vi "市电监测-自动重合闸.vi"() -> ()   [LabVIEW 2016, in "环境动力监测库.lvlib" / "自动重合闸库.lvlib"]
uses:
  <vilib>/Utility/miscctls.llb/LVPointTypeDef.ctl
  <vilib>/ptbypt/NI_PtbyPt.lvlib
  <vilib>/Utility/config.llb/NI_LVConfig.lvlib
panel:
  in  "解除告警":bool
  out "日用电量":dbl caption="日用电量：" format="%#.1f"
  out "小时用电量":dbl caption="小时用电量：" format="%#.1f"
  in  "清零":bool
  out "累计用电量":dbl caption="累计用电量：" format="%#.1f"
  out "漏电报警累加值":u16 caption="漏电报警次数："
  out "当前报警状态":u16(ring) caption="当前报警状态：" items=["无报警"=0, "过压报警"=1, "欠压报警"=2, "过流报警"=4, "漏电报警"=8]
  out "通讯状态":u16(ring) caption="通讯状态：" items=["正常", "异常"]
  out "过流报警累加值":u16 caption="过流报警次数："
  out "欠压报警累加值":u16 caption="欠压报警次数："
  out "过压报警累加值":u16 caption="过压报警次数："
  out "当前漏电电流":dbl caption="当前漏电电流："
  out "当前电流":dbl caption="当前电流："
  out "当前电压":u16 caption="当前电压："
  # "市电监测/自动重合闸"
  # "KW·h"
  # "KW·h"
  # "KW·h"
  # "mA"
  # "A"
  # "V"
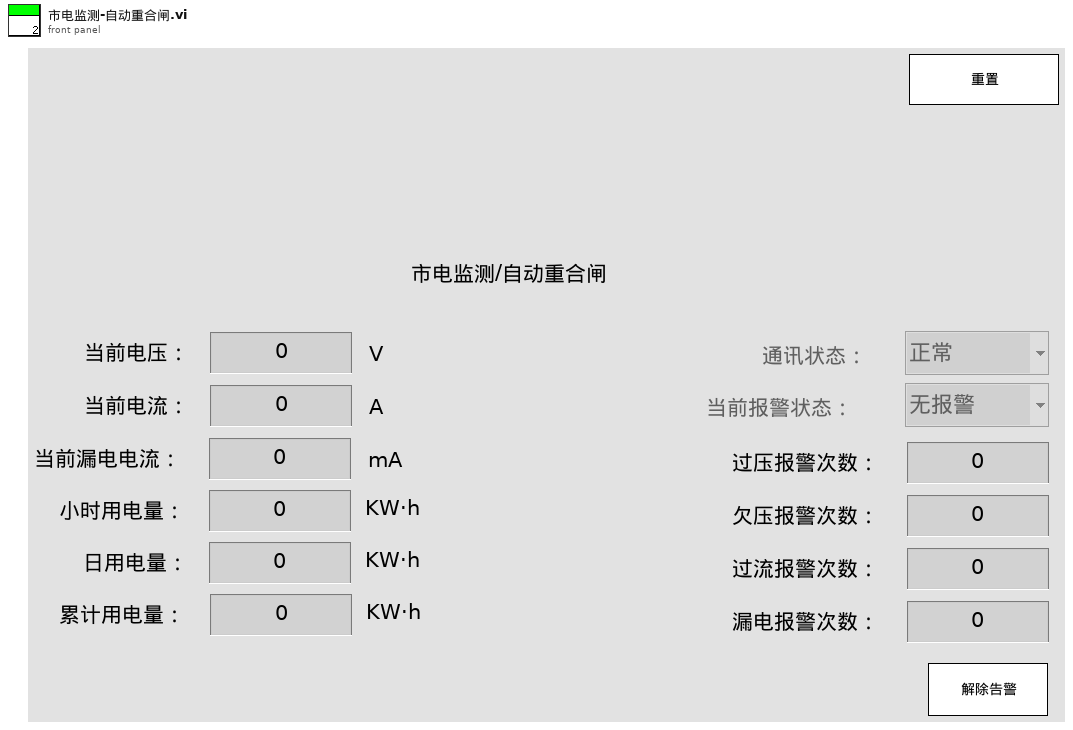
[diagram p1: front panel]
types:
  T1 = typedef "LVPointTypeDef.ctl" = cluster{"Horizontal":i16, "Vertical":i16}
  T2 = typedef "NI_LVConfig.lvlib/Config Data RefNum.ctl" = refnum<k1>
  T3 = cluster{"时间标识":timestamp, "设备":string, "日志信息":string}
  T4 = cluster{"状态":cluster{"R0":i16, "R1":i16, "R2":i16, "R3":i16, "R4":i16, "R5":i16, "R6":i16, "R7":i16, "R8":i16, "R9":i16, "R10":i16, "R11":i16, "R12":i16, "R13":i16, "R14":i16, "R15":i16, "R16":i16, "R17":i16, "R18":i16, "R19":i16, "R20":i16, "R21":i16, "R22":i16, "R23":i16, "R24":i16, "R25":i16, "R26":i16, "R27":i16, "R28":i16, "R29":i16, "R30":i16, "R31":i16, "R32":i16, "R33":i16, "R34":i16, "R35":i16, "R36":i16, "R37":i16, "R38":i16, "R39":i16}, "输入状态":bool[], "输出状态":bool[], "参数设置":cluster{"R100":i16, "R101":i16, "R102":i16, "R103":i16, "R104":i16, "R105":i16, "R106":i16, "R107":i16, "R108":i16, "R109":i16, "R110":i16, "R111":i16, "R112":i16, "R113":i16, "R114":i16, "R115":i16, "R116":i16, "R117":i16, "R118":i16, "R119":i16, "R120":i16, "R121":i16, "R122":i16, "R123":i16}, "转换值":cluster{"AD0":sgl, "AD1":sgl, "AD2":sgl, "AD3":sgl, "AD4":sgl, "AD5":sgl}}
  T5 = cluster{"R0":i16, "R1":i16, "R2":i16, "R3":i16, "R4":i16, "R5":i16, "R6":i16, "R7":i16, "R8":i16, "R9":i16, "R10":i16, "R11":i16, "R12":i16, "R13":i16, "R14":i16, "R15":i16, "R16":i16, "R17":i16, "R18":i16, "R19":i16, "R20":i16, "R21":i16, "R22":i16, "R23":i16, "R24":i16, "R25":i16, "R26":i16, "R27":i16, "R28":i16, "R29":i16, "R30":i16, "R31":i16, "R32":i16, "R33":i16, "R34":i16, "R35":i16, "R36":i16, "R37":i16, "R38":i16, "R39":i16}
  T6 = cluster{"状态":cluster{"R0":i16, "R1":i16, "R2":i16, "R3":i16, "R4":i16, "R5":i16, "R6":i16, "R7":i16, "R8":i16, "R9":i16, "R10":i16, "R11":i16, "R12":i16, "R13":i16, "R14":i16, "R15":i16, "R16":i16, "R17":i16, "R18":i16, "R19":i16, "R20":i16, "R21":i16, "R22":i16, "R23":i16, "R24":i16, "R25":i16, "R26":i16, "R27":i16, "R28":i16, "R29":i16, "R30":i16, "R31":i16, "R32":i16, "R33":i16, "R34":i16, "R35":i16, "R36":i16, "R37":i16, "R38":i16, "R39":i16, "R40":i16, "R41":i16, "R42":i16, "R43":i16, "R44":i16, "R45":i16, "R46":i16, "R47":i16, "R48":i16, "R49":i16, "R50":i16, "R51":i16, "R52":i16, "R53":i16, "R54":i16, "R55":i16, "R56":i16, "R57":i16, "R58":i16, "R59":i16, "R60":i16, "R61":i16, "R62":i16, "R63":i16, "R64":i16, "R65":i16, "R66":i16, "R67":i16, "R68":i16, "R69":i16}, "输入状态":bool[], "输出状态":bool[], "报警簇":bool[], "参数设置":cluster{"R100":i16, "R101":i16, "R102":i16, "R103":i16, "R104":i16, "R105":i16, "R106":i16, "R107":i16, "R108":i16, "R109":i16, "R110":i16, "R111":i16, "R112":i16, "R113":i16, "R114":i16, "R115":i16, "R116":i16, "R117":i16, "R118":i16, "R119":i16, "R120":i16, "R121":i16, "R122":i16, "R123":i16, "R124":i16}, "转换值":cluster{"AD0":sgl, "AD1":sgl, "AD2":sgl, "AD3":sgl, "AD4":sgl, "AD5":sgl}, "看门狗启用":bool, "氨氮模块名称":string, "总磷模块名称":string}
  T7 = cluster{"R0":i16, "R1":i16, "R2":i16, "R3":i16, "R4":i16, "R5":i16, "R6":i16, "R7":i16, "R8":i16, "R9":i16, "R10":i16, "R11":i16, "R12":i16, "R13":i16, "R14":i16, "R15":i16, "R16":i16, "R17":i16, "R18":i16, "R19":i16, "R20":i16, "R21":i16, "R22":i16, "R23":i16, "R24":i16, "R25":i16, "R26":i16, "R27":i16, "R28":i16, "R29":i16, "R30":i16, "R31":i16, "R32":i16, "R33":i16, "R34":i16, "R35":i16, "R36":i16, "R37":i16, "R38":i16, "R39":i16, "R40":i16, "R41":i16, "R42":i16, "R43":i16, "R44":i16, "R45":i16, "R46":i16, "R47":i16, "R48":i16, "R49":i16, "R50":i16, "R51":i16, "R52":i16, "R53":i16, "R54":i16, "R55":i16, "R56":i16, "R57":i16, "R58":i16, "R59":i16, "R60":i16, "R61":i16, "R62":i16, "R63":i16, "R64":i16, "R65":i16, "R66":i16, "R67":i16, "R68":i16, "R69":i16}
  T8 = cluster{"漏水监测输出":cluster{"漏水监测告警":bool, "告警内容":string}, "门禁监测输出":cluster{"门禁监测告警":bool, "告警内容":string}, "门禁监测输出2":cluster{"门禁监测告警":bool, "告警内容":string}, "温湿度监测输出":cluster{"温湿度监测告警":bool, "告警内容":string}, "烟雾监测输出":cluster{"烟雾监测告警":bool, "告警内容":string}, "空调监测输出":cluster{"空调监测告警":bool, "告警内容":string}, "自动重合闸输出":cluster{"自动重合闸告警":bool, "告警内容":string}, "红外入侵输出":cluster{"红外入侵告警":bool, "告警内容":string}, "振动输出":cluster{"振动告警":bool, "告警内容":string}, "UPS输出":cluster{"UPS告警":bool, "告警内容":string}, "蓄电池输出":cluster{"蓄电池告警":bool, "告警内容":string}, "蓄电池输出2":cluster{"蓄电池告警":bool, "告警内容":string}, "GPS输出":cluster{"定位告警":bool, "告警内容":string}, "北斗输出":cluster{"定位告警":bool, "告警内容":string}, "气象输出":cluster{"气象告警":bool, "告警内容":string}}
  T9 = cluster{"市电":cluster{"状态":bool, "电压:":u16, "电流：":dbl, "详情  ":bool}, "UPS":cluster{"状态":bool, "输入电压:":sgl, "输出电压:":sgl, "电池电量:":u8, "电量":u16, "详情  ":bool}, "蓄电池12V":cluster{"状态":bool, "电压:":sgl, "电流:":sgl, "电池电量:":u8, "电量":u16, "详情  ":bool}, "蓄电池24V":cluster{"状态":bool, "电压:":sgl, "电流:":sgl, "电池电量:":u8, "电量":u16, "详情  ":bool}}
  T10 = cluster{"时间标识":timestamp, "测量模式":string, "数据类型":string, "监测值":sgl, "单位":string, "数据标识":string, "因子编码":string}
  T11 = typedef "LVDateTimeRec.ctl" = cluster{"秒数的小数部分":dbl, "秒":i32, "分":i32, "时":i32, "日":i32, "月":i32, "年":i32, "天数（周）":i32, "天数（年）":i32, "DST":i32}
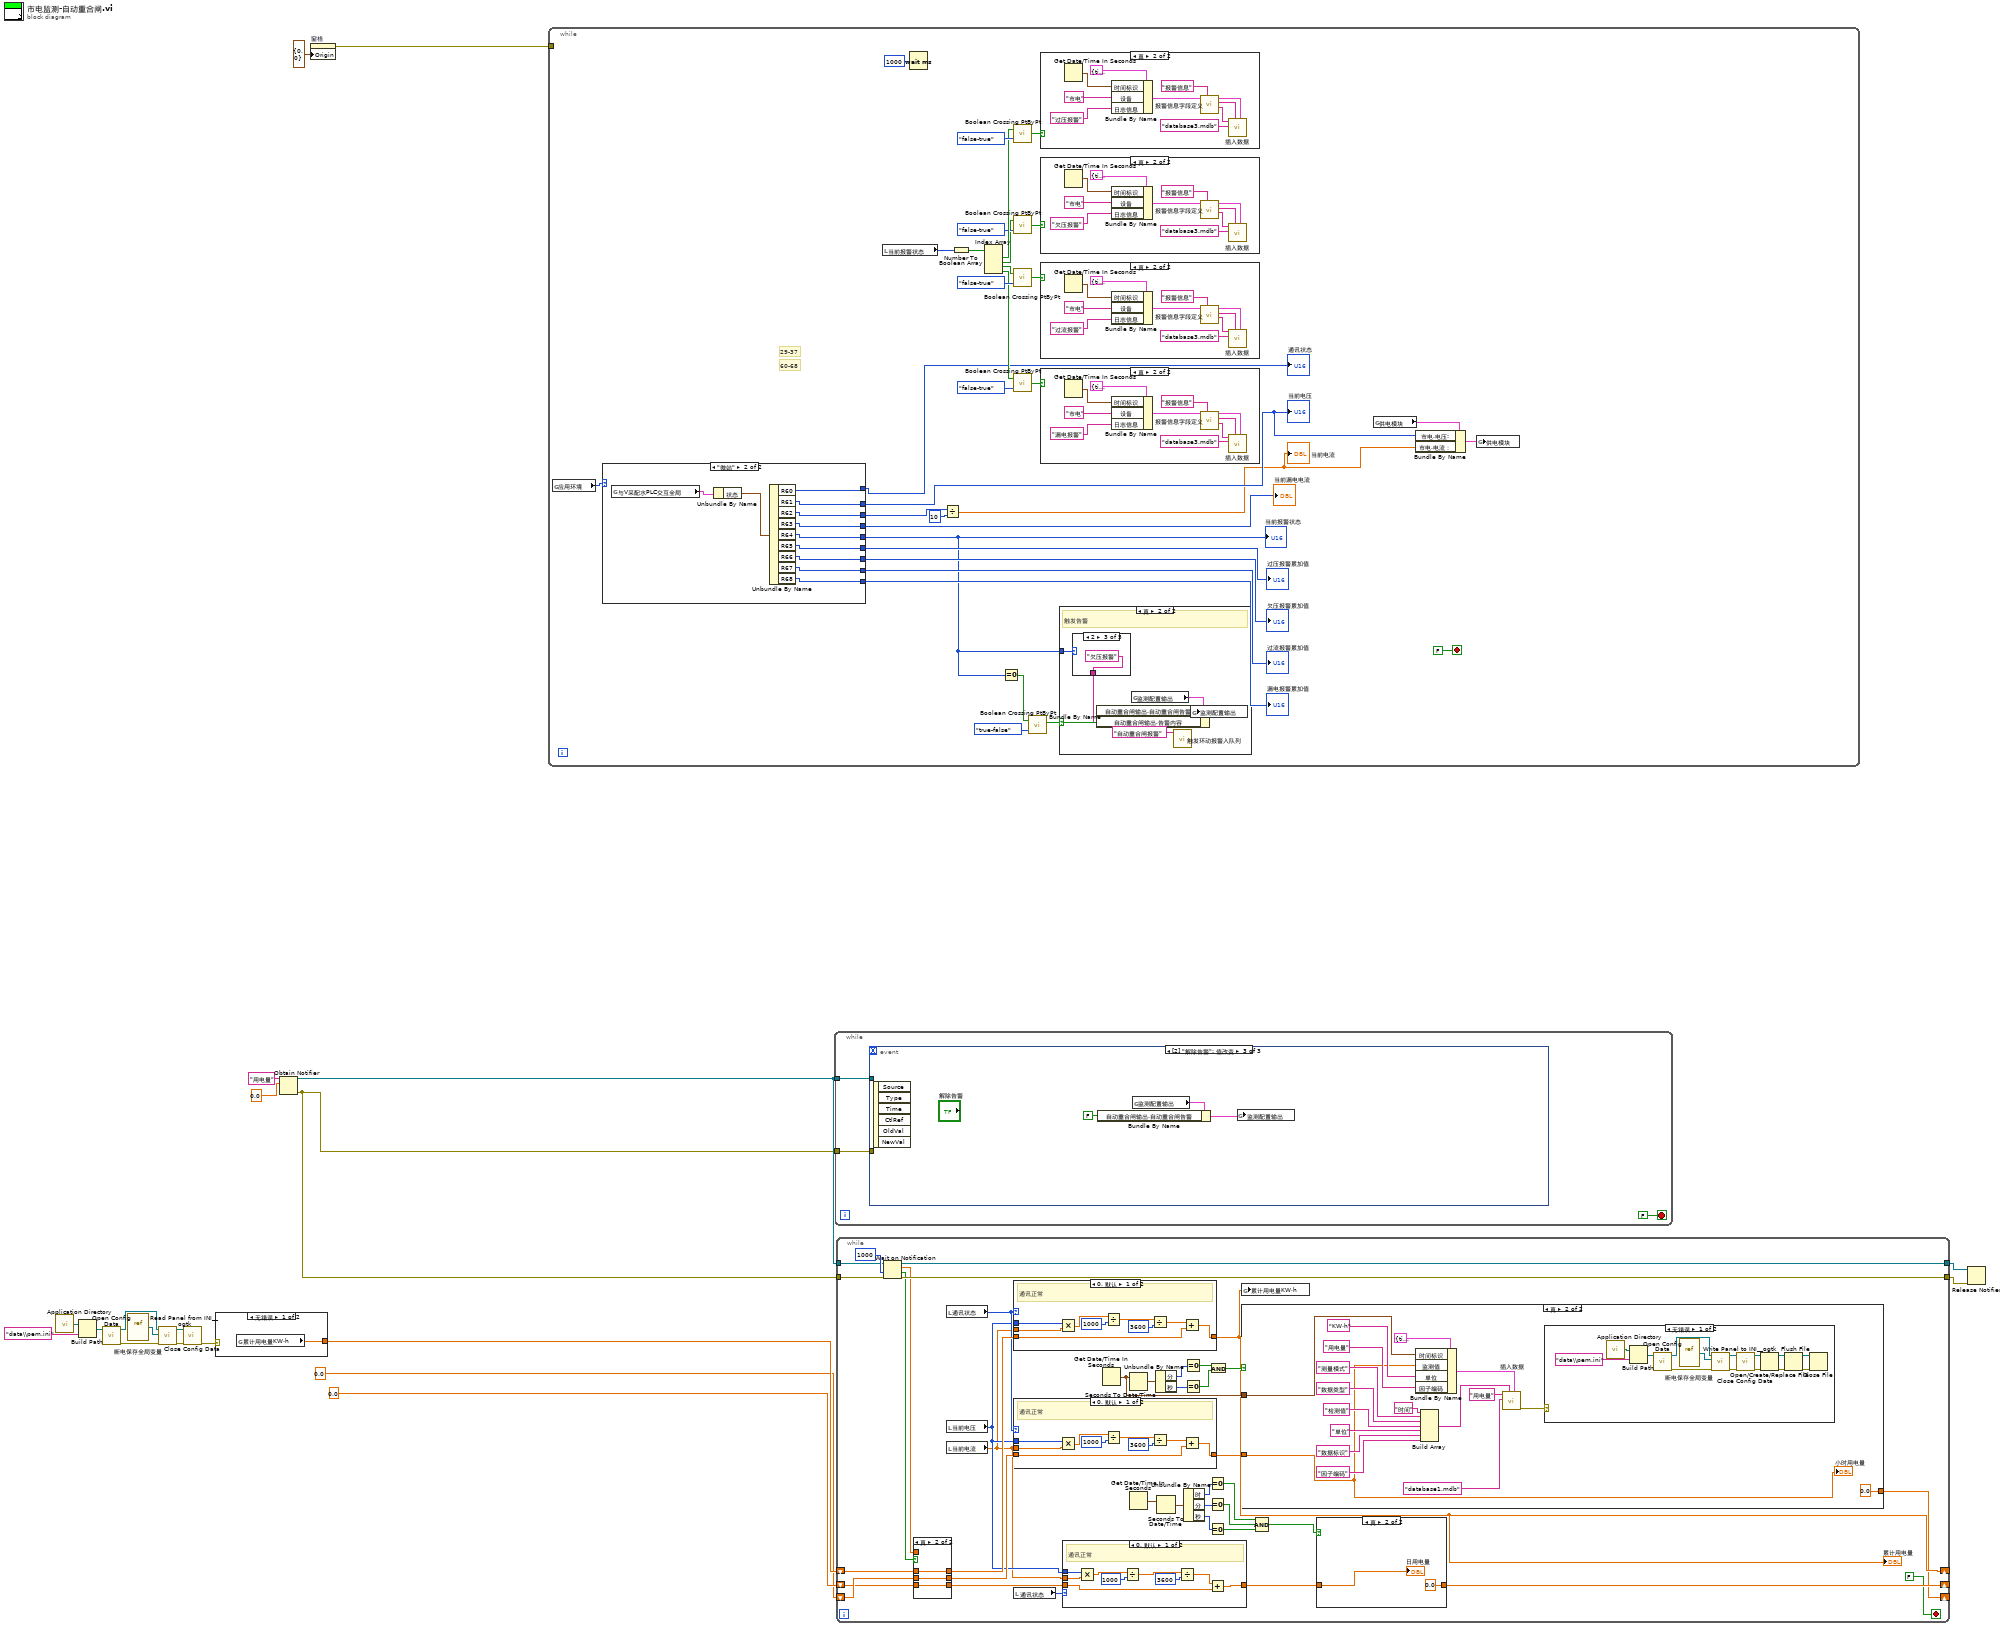
[diagram p0: block diagram]
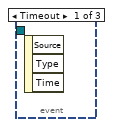
[diagram p9: hidden frame]
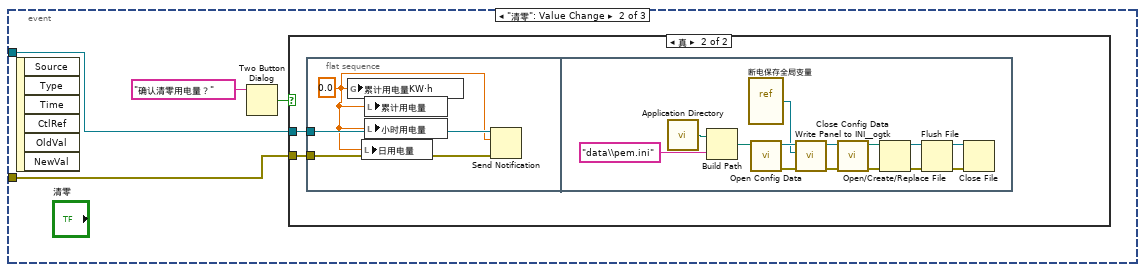
[diagram p10: hidden frame]
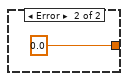
[diagram p12: hidden frame]
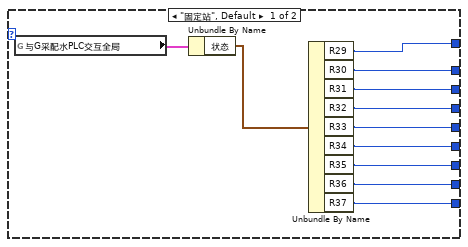
[diagram p13: hidden frame]
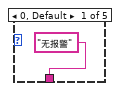
[diagram p15: hidden frame]
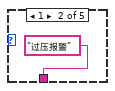
[diagram p16: hidden frame]
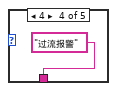
[diagram p17: hidden frame]
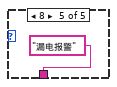
[diagram p18: hidden frame]
diagram:
  n1 = call <vilib>:"Application Directory.vi"() -> ("Application Directory"=w18:path)
  n2 = Build Path(base path=w18, name or relative path="data\\pem.ini" ("名称或相对路径")) -> (appended path=w16:path)
  n3 = call <vilib>:"Open Config Data.vi"("configuration file path"=w16) -> ("error out"=w12:errorcluster, "refnum"=w15:T2)  [unwired: 8 in, 1 out]
  n4 = vi-ref "断电保存全局变量.vi"() -> (w14:refnum<vi>)
  n5 = call <userlib>:"Read Panel from INI__ogtk.vi"("error in (no error)"=w12, "VI ref"=w14, "refnum"=w15) -> ("error out"=w11:errorcluster, "refnum out"=w13:T2)  [unwired: 7 in]
  n6 = call <vilib>:"Close Config Data.vi"("error in (no error)"=w11, "refnum"=w13) -> ("error out"=w10:errorcluster)  [unwired: 8 in, 1 out]
  n7 = case shown="无错误" w10 {
    tunnel: [w21 0.0 ("累计用电量KW/h")] -> w3
    frame No Error {
      n8 = global read "断电保存全局变量.vi" "累计用电量KW·h"() -> (w21:dbl)
    }
    frame Error {
    }
  }
  n9 = Obtain Notifier(name (unnamed)="用电量" ("名称（未命名）"), notification data type=0.0 ("y")) -> (notifier out=w7:refnum<notifier>, error out=w6:errorcluster)  [unwired: 2 in, 1 out]
  n10 = property on="窗格" class="Pane"("Origin"=T1 {"Horizontal"=0, "Vertical"=0} ("原点")) -> (error out=w19:errorcluster)  [unwired: 2 in, 1 out]
  n11 = while {
    tunnel: w19 -> [_]
    stop <- FALSE stop-if-true
    # "60-68"
    # "29-37"
    n12 = global read "外部交互全局变量.vi" "应用环境"() -> (w36:enum16{"固定站", "微站", "浮标", "浮船"})
    n13 = case shown="\"微站\"" w36 {
      tunnel: [w64 w75] -> w35
      tunnel: [w63 w74] -> w25
      tunnel: [w62 w73] -> w34
      tunnel: [w61 w72] -> w33
      tunnel: [w60 w71] -> w23
      tunnel: [w59 w70] -> w32
      tunnel: [w58 w69] -> w31
      tunnel: [w57 w68] -> w30
      tunnel: [w56 w67] -> w29
      frame "固定站", Default {
        n14 = global read "外部交互全局变量.vi" "与G采配水PLC交互全局"() -> (w66:T4)
        n15 = Unbundle By Name(w66) -> ("状态"=w65:T5)
        n16 = Unbundle By Name(w65) -> ("R29"=w64:i16, "R30"=w63:i16, "R31"=w62:i16, "R32"=w61:i16, "R33"=w60:i16, "R34"=w59:i16, "R35"=w58:i16, "R36"=w57:i16, "R37"=w56:i16)
      }
      frame "微站" {
        n17 = global read "外部交互全局变量.vi" "与V采配水PLC交互全局"() -> (w77:T6)
        n18 = Unbundle By Name(w77) -> ("状态"=w76:T7)
        n19 = Unbundle By Name(w76) -> ("R60"=w75:i16, "R61"=w74:i16, "R62"=w73:i16, "R63"=w72:i16, "R64"=w71:i16, "R65"=w70:i16, "R66"=w69:i16, "R67"=w68:i16, "R68"=w67:i16)
      }
    }
    "通讯状态" <- w35
    "当前电压" <- w25
    "当前漏电电流" <- w33
    "当前报警状态" <- w23
    "过压报警累加值" <- w32
    "欠压报警累加值" <- w31
    "过流报警累加值" <- w30
    "漏电报警累加值" <- w29
    n20 = local read "当前报警状态"() -> (w54:u16)
    n21 = Wait (ms)(milliseconds to wait=u32 1000 ("等待时间（毫秒）")) -> ()  [unwired: 1 out]
    n22 = Divide(x=w34, y=i16 10) -> (x/y=w24:dbl)
    "当前电流" <- w24
    n23 = Number To Boolean Array(number=w54) -> (Boolean array=w53:bool[])
    n24 = Index Array(array=w53) -> (element #1=w51:bool, element #2=w45:bool, element #3=w44:bool, element #4=w41:bool)  [unwired: 4 in]
    n25 = Equal To 0?(x=w23) -> (x = 0?=w37:bool)
    n26 = call <vilib>:"Boolean Crossing PtByPt.vi"("direction"=enum16{"either", "false-true", "true-false"}."false-true", "input"=w51) -> ("crossing"=w50:bool)  [unwired: 1 in]
    n27 = call <vilib>:"Boolean Crossing PtByPt.vi"("direction"=enum16{"either", "false-true", "true-false"}."false-true", "input"=w45) -> ("crossing"=w49:bool)  [unwired: 1 in]
    n28 = call <vilib>:"Boolean Crossing PtByPt.vi"("direction"=enum16{"either", "false-true", "true-false"}."false-true", "input"=w44) -> ("crossing"=w46:bool)  [unwired: 1 in]
    n29 = call <vilib>:"Boolean Crossing PtByPt.vi"("direction"=enum16{"either", "false-true", "true-false"}."false-true", "input"=w41) -> ("crossing"=w43:bool)  [unwired: 1 in]
    n30 = call <vilib>:"Boolean Crossing PtByPt.vi"("direction"=enum16{"either", "false-true", "true-false"}."true-false", "input"=w37) -> ("crossing"=w28:bool)  [unwired: 1 in]
    n31 = case shown="真" w50 {
      frame False {
      }
      frame True {
        n32 = Get Date/Time In Seconds() -> (seconds since 1Jan1904=w127:timestamp)
        n33 = Bundle By Name(cluster=T3 {"时间标识"=timestamp(0 s since 1904-01-01), "设备"="", "日志信息"=""} ("data in"), "时间标识"=w127, "设备"="市电", "日志信息"="过压报警") -> (w126:T3)
        n34 = call "报警信息字段定义.vi"("table输入"="报警信息", "data in"=w126) -> ("table输出"=w122:string, "columns"=w121:string[], "data out"=w120:T3)  [unwired: 7 in]
        n35 = call "插入数据.vi"("data"=w120, "columns"=w121, "database"="database3.mdb", "table"=w122) -> ()  [unwired: 7 in, 1 out]
      }
    }
    n36 = case shown="真" w49 {
      frame False {
      }
      frame True {
        n37 = Get Date/Time In Seconds() -> (seconds since 1Jan1904=w117:timestamp)
        n38 = Bundle By Name(cluster=T3 {"时间标识"=timestamp(0 s since 1904-01-01), "设备"="", "日志信息"=""} ("data in"), "时间标识"=w117, "设备"="市电", "日志信息"="欠压报警") -> (w116:T3)
        n39 = call "报警信息字段定义.vi"("table输入"="报警信息", "data in"=w116) -> ("table输出"=w112:string, "columns"=w111:string[], "data out"=w110:T3)  [unwired: 7 in]
        n40 = call "插入数据.vi"("data"=w110, "columns"=w111, "database"="database3.mdb", "table"=w112) -> ()  [unwired: 7 in, 1 out]
      }
    }
    n41 = case shown="真" w46 {
      frame False {
      }
      frame True {
        n42 = Get Date/Time In Seconds() -> (seconds since 1Jan1904=w107:timestamp)
        n43 = Bundle By Name(cluster=T3 {"时间标识"=timestamp(0 s since 1904-01-01), "设备"="", "日志信息"=""} ("data in"), "时间标识"=w107, "设备"="市电", "日志信息"="过流报警") -> (w106:T3)
        n44 = call "报警信息字段定义.vi"("table输入"="报警信息", "data in"=w106) -> ("table输出"=w102:string, "columns"=w101:string[], "data out"=w100:T3)  [unwired: 7 in]
        n45 = call "插入数据.vi"("data"=w100, "columns"=w101, "database"="database3.mdb", "table"=w102) -> ()  [unwired: 7 in, 1 out]
      }
    }
    n46 = case shown="真" w43 {
      frame False {
      }
      frame True {
        n47 = Get Date/Time In Seconds() -> (seconds since 1Jan1904=w97:timestamp)
        n48 = Bundle By Name(cluster=T3 {"时间标识"=timestamp(0 s since 1904-01-01), "设备"="", "日志信息"=""} ("data in"), "时间标识"=w97, "设备"="市电", "日志信息"="漏电报警") -> (w96:T3)
        n49 = call "报警信息字段定义.vi"("table输入"="报警信息", "data in"=w96) -> ("table输出"=w92:string, "columns"=w91:string[], "data out"=w90:T3)  [unwired: 7 in]
        n50 = call "插入数据.vi"("data"=w90, "columns"=w91, "database"="database3.mdb", "table"=w92) -> ()  [unwired: 7 in, 1 out]
      }
    }
    n51 = case shown="真" w28 {
      selector: w28 -> [_ w80]
      tunnel: w23 -> [_ w79]
      frame False {
      }
      frame True {
        # "触发告警"
        n52 = case shown="2" w79 {
          tunnel: ["无报警" ("日志信息") "过压报警" ("日志信息") "欠压报警" ("日志信息") "过流报警" ("日志信息") "漏电报警" ("日志信息")] -> w78
          frame 0, Default {
          }
          frame 1 {
          }
          frame 2 {
          }
          frame 4 {
          }
          frame 8 {
          }
        }
        n53 = global read "断电保存全局变量.vi" "监测配置输出"() -> (w81:T8)
        n54 = Bundle By Name(cluster=w81, "自动重合闸输出.自动重合闸告警"=w80, "自动重合闸输出.告警内容"=w78) -> (w82:T8)
        n55 = call "触发环动报警入队列.vi"("报警内容"="自动重合闸报警") -> ()  [unwired: 11 in]
        n56 = global write "断电保存全局变量.vi" "监测配置输出"(w82) -> ()
      }
    }
    n57 = global read "内部交互全局变量.vi" "供电模块"() -> (w27:T9)
    n58 = Bundle By Name(cluster=w27, "市电.电压:"=w25, "市电.电流："=w24) -> (w26:T9)
    n59 = global write "内部交互全局变量.vi" "供电模块"(w26) -> ()
  }
  n60 = while {
    tunnel: w7 -> [w131]
    tunnel: w6 -> [w130]
    stop <- FALSE stop-if-true
    n61 = event shown="[2] \"解除告警\": 值改变" {
      selector: _ -> [_ _ _]
      dyn-events: _ -> [_ _ _]
      timeout: _ -> [_ _ _]
      tunnel: w131 -> [_ w133 _]
      tunnel: w130 -> [_ w132 _]
      event Timeout {
        n62 = event-data() -> ()  [unwired: 1 in, 3 out]
      }
      event "清零": Value Change {
        n63 = event-data() -> ()  [unwired: 1 in, 6 out]
        n64 = Two Button Dialog(message="确认清零用电量？" ("消息")) -> (T button?=w134:bool)  [unwired: 2 in]
        n65 = case shown="真" w134 {
          tunnel: w133 -> [_ w137]
          tunnel: w132 -> [_ w136]
          frame False {
          }
          frame True {
            n66 = flat-sequence {
              tunnel: w137 -> [w140]
              tunnel: w136 -> [w139]
              frame #0 {
                w138 = 0.0 ("累计用电量KW/h")
                n67 = global write "断电保存全局变量.vi" "累计用电量KW·h"(w138) -> ()
                n68 = local write "日用电量"(w138) -> ()
                n69 = local write "累计用电量"(w138) -> ()
                n70 = local write "小时用电量"(w138) -> ()
                n71 = Send Notification(notification=w138, notifier=w140, error in (no error)=w139) -> ()  [unwired: 2 out]
              }
              frame #1 {
                n72 = call <vilib>:"Application Directory.vi"() -> ("Application Directory"=w143:path)
                n73 = Build Path(base path=w143, name or relative path="data\\pem.ini" ("名称或相对路径")) -> (appended path=w144:path)
                n74 = vi-ref "断电保存全局变量.vi"() -> (w141:refnum<vi>)
                n75 = call <vilib>:"Open Config Data.vi"("configuration file path"=w144) -> ("error out"=w147:errorcluster, "refnum"=w145:T2)  [unwired: 8 in, 1 out]
                n76 = call <userlib>:"Write Panel to INI__ogtk.vi"("error in (no error)"=w147, "VI ref"=w141, "refnum"=w145) -> ("error out"=w148:errorcluster, "refnum out"=w146:T2)  [unwired: 7 in]
                n77 = call <vilib>:"Close Config Data.vi"("error in (no error)"=w148, "refnum"=w146) -> ("error out"=w153:errorcluster, "file path"=w154:path)  [unwired: 8 in]
                n78 = Open/Create/Replace File(file path (use dialog)=w154, error in=w153) -> (refnum out=w150:refnum<file>, error out=w149:errorcluster)  [unwired: 4 in, 1 out]
                n79 = Flush File(refnum=w150, error in=w149) -> (refnum out=w151:refnum<file>, error out=w152:errorcluster)
                n80 = Close File(refnum=w151, error in=w152) -> ()  [unwired: 2 out]
              }
            }
          }
        }
      }
      event "解除告警": Value Change {
        n81 = event-data() -> ()  [unwired: 1 in, 6 out]
        n82 = global read "断电保存全局变量.vi" "监测配置输出"() -> (w156:T8)
        n83 = Bundle By Name(cluster=w156, "自动重合闸输出.自动重合闸告警"=FALSE) -> (w157:T8)
        n84 = global write "断电保存全局变量.vi" "监测配置输出"(w157) -> ()
      }
    }
  }
  n85 = while {
    tunnel: w7 -> [w195]
    tunnel: w6 -> [w194]
    tunnel: [w193] -> w5
    tunnel: [w192] -> w4
    shift-right: [w164] -> _
    shift-left: w3 -> [w191]
    shift-right: [w169] -> _
    shift-left: 0.0 -> [w166]
    shift-right: [w163] -> _
    shift-left: 0.0 -> [w167]
    stop <- FALSE stop-if-true
    n86 = Wait on Notification(notifier=w195, timeout in ms (-1)=1000 ("超时毫秒(-1)"), error in (no error)=w194) -> (notifier out=w193:refnum<notifier>, notification=w190:dbl, timed out?=w189:bool, error out=w192:errorcluster)  [unwired: 1 in]
    n87 = case shown="真" w189 {
      tunnel: [w263 w266] -> w188
      tunnel: w191 -> [_ w266]
      tunnel: [w263 w265] -> w161
      tunnel: w190 -> [w263 _]
      tunnel: w167 -> [_ w265]
      tunnel: w166 -> [_ w264]
      tunnel: [w263 w264] -> w165
      frame False {
      }
      frame True {
      }
    }
    n88 = local read "通讯状态"() -> (w160:u16)
    n89 = local read "当前电压"() -> (w159:u16)
    n90 = local read "当前电流"() -> (w158:dbl)
    n91 = case shown="0, 默认" w160 {
      tunnel: w159 -> [w259 _]
      tunnel: w158 -> [w258 _]
      tunnel: w188 -> [w257 w262]
      tunnel: [w256 w262] -> w164
      frame 0, Default {
        # "通讯正常"
        n92 = Multiply(x=w259, y=w258) -> (x*y=w260:dbl)
        n93 = Divide(x=w260, y=1000) -> (x/y=w254:dbl)
        n94 = Divide(x=w254, y=3600) -> (x/y=w253:dbl)
        n95 = Add(x=w253, y=w257) -> (x+y=w256:dbl)
      }
      frame 1 {
        # "通信异常"
      }
    }
    "累计用电量" <- w164
    n96 = case shown="0, 默认" w160 {
      tunnel: w159 -> [w203 _]
      tunnel: w158 -> [w202 _]
      tunnel: w161 -> [w201 w206]
      tunnel: [w200 w206] -> w162
      frame 0, Default {
        # "通讯正常"
        n97 = Multiply(x=w203, y=w202) -> (x*y=w204:dbl)
        n98 = Divide(x=w204, y=1000) -> (x/y=w198:dbl)
        n99 = Divide(x=w198, y=3600) -> (x/y=w197:dbl)
        n100 = Add(x=w197, y=w201) -> (x+y=w200:dbl)
      }
      frame 1 {
        # "通信异常"
      }
    }
    n101 = local read "通讯状态"() -> (w172:u16)
    n102 = case shown="0, 默认" w172 {
      tunnel: w159 -> [w216 _]
      tunnel: w158 -> [w215 _]
      tunnel: w165 -> [w214 w219]
      tunnel: [w213 w219] -> w170
      frame 0, Default {
        # "通讯正常"
        n103 = Multiply(x=w216, y=w215) -> (x*y=w217:dbl)
        n104 = Divide(x=w217, y=1000) -> (x/y=w211:dbl)
        n105 = Divide(x=w211, y=3600) -> (x/y=w210:dbl)
        n106 = Add(x=w210, y=w214) -> (x+y=w213:dbl)
      }
      frame 1 {
        # "通信异常"
      }
    }
    n107 = Get Date/Time In Seconds() -> (seconds since 1Jan1904=w181:timestamp)
    n108 = Seconds To Date/Time(time stamp (now)=w181) -> (date time rec=w183:T11)  [unwired: 1 in]
    n109 = Get Date/Time In Seconds() -> (seconds since 1Jan1904=w180:timestamp)
    n110 = Unbundle By Name(w183) -> ("分"=w184:i32, "秒"=w185:i32)
    n111 = Seconds To Date/Time(time stamp (now)=w180) -> (date time rec=w179:T11)  [unwired: 1 in]
    n112 = Unbundle By Name(w179) -> ("时"=w174:i32, "分"=w178:i32, "秒"=w177:i32)
    n113 = Equal To 0?(x=w184) -> (x = 0?=w186:bool)
    n114 = Equal To 0?(x=w185) -> (x = 0?=w187:bool)
    n115 = Equal To 0?(x=w174) -> (x = 0?=w173:bool)
    n116 = Equal To 0?(x=w178) -> (x = 0?=w176:bool)
    n117 = Equal To 0?(x=w177) -> (x = 0?=w175:bool)
    n118 = And(x=w186, y=w187) -> (x .and. y?=w182:bool)
    n119 = global write "断电保存全局变量.vi" "累计用电量KW·h"(w164) -> ()
    n120 = case shown="真" w182 {
      tunnel: [w220 0.0 ("y")] -> w163
      tunnel: w162 -> [w220 w222]
      tunnel: w181 -> [_ w235]
      frame False {
      }
      frame True {
        n121 = Bundle By Name(cluster=T10 {"时间标识"=timestamp(0 s since 1904-01-01), "测量模式"="水样测试", "数据类型"="N", "监测值"=0.0, "单位"="mg/L", "数据标识"="N", "因子编码"=""} ("data"), "时间标识"=w235, "监测值"=w222, "单位"="KW·h", "因子编码"="用电量") -> (w223:T10)
        n122 = Build Array("时间", "测量模式", "数据类型", "检测值", "单位", "数据标识", "因子编码") -> (w224:string[])
        n123 = call "插入数据.vi"("data"=w223, "columns"=w224, "database"="database1.mdb", "table"="用电量") -> ("error out"=w227:errorcluster)  [unwired: 7 in]
        n124 = case shown="无错误" w227 {
          frame No Error {
            n125 = call <vilib>:"Application Directory.vi"() -> ("Application Directory"=w241:path)
            n126 = Build Path(base path=w241, name or relative path="data\\pem.ini" ("名称或相对路径")) -> (appended path=w242:path)
            n127 = call <vilib>:"Open Config Data.vi"("configuration file path"=w242) -> ("error out"=w245:errorcluster, "refnum"=w243:T2)  [unwired: 8 in, 1 out]
            n128 = vi-ref "断电保存全局变量.vi"() -> (w239:refnum<vi>)
            n129 = call <userlib>:"Write Panel to INI__ogtk.vi"("error in (no error)"=w245, "VI ref"=w239, "refnum"=w243) -> ("error out"=w246:errorcluster, "refnum out"=w244:T2)  [unwired: 7 in]
            n130 = call <vilib>:"Close Config Data.vi"("error in (no error)"=w246, "refnum"=w244) -> ("error out"=w251:errorcluster, "file path"=w252:path)  [unwired: 8 in]
            n131 = Open/Create/Replace File(file path (use dialog)=w252, error in=w251) -> (refnum out=w248:refnum<file>, error out=w247:errorcluster)  [unwired: 4 in, 1 out]
            n132 = Flush File(refnum=w248, error in=w247) -> (refnum out=w249:refnum<file>, error out=w250:errorcluster)
            n133 = Close File(refnum=w249, error in=w250) -> ()  [unwired: 2 out]
          }
          frame Error {
          }
        }
        "小时用电量" <- w222
      }
    }
    n134 = Compound Arithmetic op=AND ("复合运算")(w173, w176, w175) -> (w171:bool)
    n135 = case shown="真" w171 {
      tunnel: w170 -> [w207 w209]
      tunnel: [w207 0.0] -> w169
      frame False {
      }
      frame True {
        "日用电量" <- w209
      }
    }
  }
  n136 = Release Notifier(notifier=w5, error in (no error)=w4) -> ()  [unwired: 1 in, 3 out]
